vi "Name.vi"(8 "error in (no error)":errorcluster, 11 "LUnit Test Suite in":refnum<class "LUnit Test Suite.lvclass">) -> (0 "error out":errorcluster, 2 "Name":string, 3 "LUnit Test Suite out":refnum<class "LUnit Test Suite.lvclass">)   [LabVIEW 2020, in "LUnit Test Suite.lvclass"]
doc: "Return name of test suite."
uses:
  LUnit Test Suite.lvclass
  LUnit Test Suite.lvclass/LUnit Test Suite.ctl
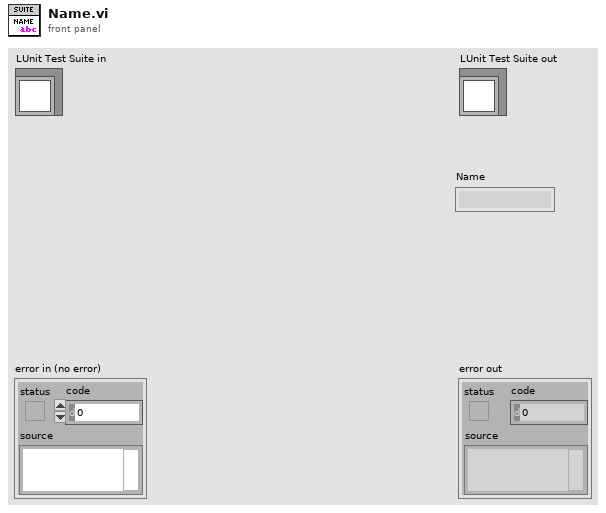
[diagram p1: front panel]
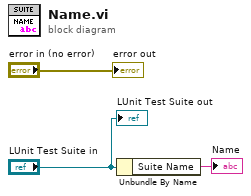
[diagram p0: block diagram]
diagram:
  n1 = Unbundle By Name("LUnit Test Suite in") -> ("Suite Name"=→"Name":string)
  "error out" <- "error in (no error)"
  "LUnit Test Suite out" <- "LUnit Test Suite in"
